vi "Grid ChangeValueCol.vi"(8 "error in (no error)":errorcluster caption="エラー入力（エラーなし）", 9 "OldVal":string[][](array[string]), 10 "NewVal":string[][](array[string]), 11 "出力クラスタ":T2) -> (0 "error out":errorcluster caption="エラー出力", 2 "編集位置":T1, 3 "変化位置配列":T1[](array[typedef]))   [LabVIEW 2014]
uses:
  Grid Parameter.ctl
  <vilib>/Utility/miscctls.llb/LVRowAndColumnTypeDef.ctl
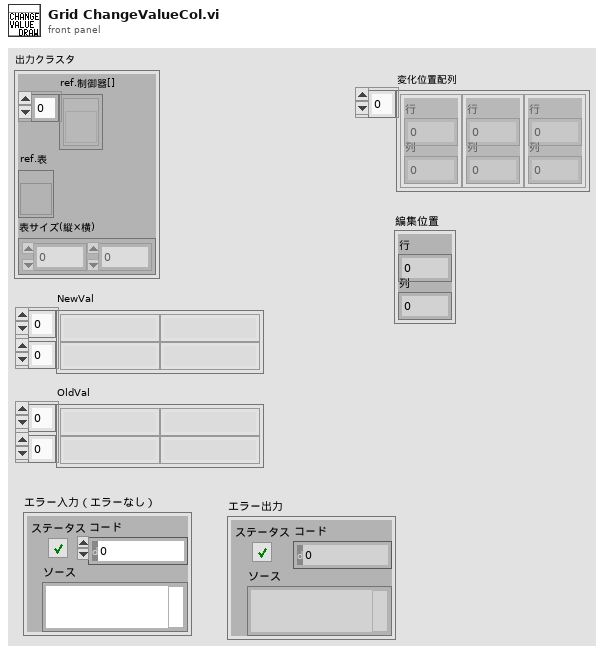
[diagram p1: front panel]
types:
  T1 = typedef "LVRowAndColumnTypeDef.ctl" = cluster{"Row":i32, "Column":i32}
  T2 = typedef "Grid Parameter.ctl" = cluster{"ref.制御器[]":refnum<vi>[], "ref.表":refnum<vi>, "表サイズ(縦×横)":i32[]}
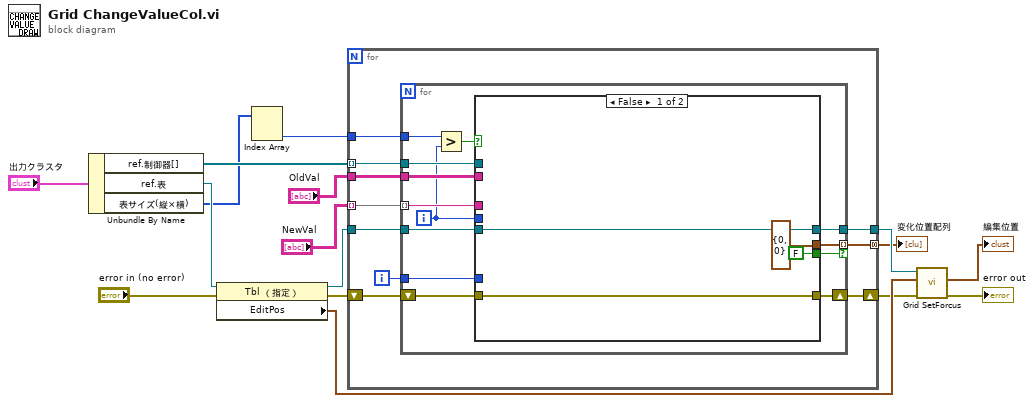
[diagram p0: block diagram]
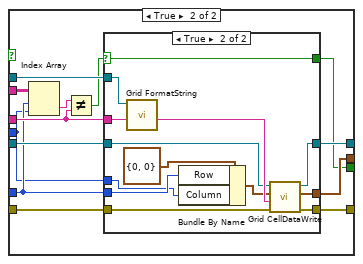
[diagram p2: hidden frame]
diagram:
  n1 = Unbundle By Name("出力クラスタ") -> ("ref.制御器[]"=w4:refnum<vi>[], "ref.表"=w16:refnum<vi>, "表サイズ(縦×横)"=w2:i32[])
  n2 = property class="Tbl （指定）"(reference=w16, error in="error in (no error)") -> (reference out=w12:refnum<vi>, error out=w3:errorcluster, "EditPos"=w14:T1)
  n3 = Index Array(array=w2) -> (element #2=w1:i32)  [unwired: 2 in, 1 out]
  n4 = for {
    tunnel: "OldVal" -> [w26]
    tunnel: "NewVal" -> [w25] mode=indexing
    tunnel: w12 -> [w23]
    tunnel: [w22] -> w13
    shift-right: [w20] -> w8
    shift-left: w3 -> [w21]
    tunnel: [w19] -> w6 mode=concatenating
    tunnel: w4 -> [w18] mode=indexing
    tunnel: w1 -> [w17]
    i -> [w24]
    n5 = for {
      tunnel: w26 -> [w35]
      tunnel: w25 -> [w38] mode=indexing
      tunnel: w24 -> [w34]
      tunnel: w18 -> [w39]
      tunnel: w23 -> [w37]
      tunnel: [w36] -> w22
      shift-right: [w32] -> w20
      shift-left: w21 -> [w33]
      tunnel: [w31] -> w19 mode=indexing if=w30
      tunnel: w17 -> [w29]
      i -> [w28]
      n6 = Greater?(x=w29, y=w28) -> (0:w27:bool)
      n7 = case shown="FALSE" w27 {
        tunnel: w39 -> [_ w56]
        tunnel: w38 -> [_ w55]
        tunnel: w37 -> [w43 w53]
        tunnel: [w43 w52] -> w36
        tunnel: w35 -> [_ w51]
        tunnel: w34 -> [_ w50]
        tunnel: w33 -> [w42 w48]
        tunnel: [w42 w47] -> w32
        tunnel: [T1 {"Row"=0, "Column"=0} ("EditPos(copy))") w46] -> w31
        tunnel: [FALSE w45] -> w30
        tunnel: w28 -> [_ w44]
        frame False {
        }
        frame True {
          n8 = Index Array(array=w51, index (row)=w50, index (col)=w44) -> (element=w49:string)
          n9 = Not Equal?(x=w49, y=w55) -> (x != y?=w54:bool)
          n10 = case shown="TRUE" w54 {
            selector: w54 -> [w57 w60]
            tunnel: w56 -> [_ w72]
            tunnel: w55 -> [_ w71]
            tunnel: w50 -> [_ w69]
            tunnel: w44 -> [_ w68]
            tunnel: w53 -> [w59 w65]
            tunnel: [w59 w64] -> w52
            tunnel: w48 -> [w58 w63]
            tunnel: [w58 w62] -> w47
            tunnel: [_ w61] -> w46
            tunnel: [w57 w60] -> w45
            frame False {
            }
            frame True {
              n11 = call "Grid FormatString.vi"("文字列"=w71, "Control入力"=w72) -> ("フォーマット後文字列"=w70:string)  [unwired: 9 in]
              n12 = Bundle By Name(cluster=T1 {"Row"=0, "Column"=0} ("EditPos"), "Row"=w69, "Column"=w68) -> (w66:T1)
              n13 = call "Grid CellDataWrite.vi"("error in (no error)"=w63, "RingText.Text"=w70, "EditPos"=w66, "Table入力"=w65) -> ("エラー出力"=w62:errorcluster, "EditPos(copy))"=w61:T1, "Table出力"=w64:refnum<vi>)  [unwired: 5 in]
            }
          }
        }
      }
    }
  }
  "変化位置配列" <- w6
  n14 = call "Grid SetForcus.vi"("エラー入力（エラーなし）"=w8, "EditPos入力"=w14, "Table入力"=w13) -> ("error out"=→"error out":errorcluster, "EditPos出力"=→"編集位置":T1)  [unwired: 6 in, 1 out]
